vi "add id.vi"(8 "error in (no error)":errorcluster, 10 "id value":variant, 11 "Cluster in":variant) -> (0 "error out":errorcluster, 3 "Cluster out":variant)   [LabVIEW 2017, in "JSONRPC Server.lvclass"]
uses:
  JSONRPC Server.lvclass
  <vilib>/National Instruments/Variant Data Manipulation/Insert Element at End.vi
  <vilib>/National Instruments/Variant Data Manipulation/Variant Data Manipulation.lvlib
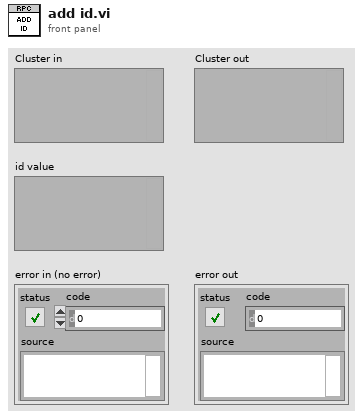
[diagram p1: front panel]
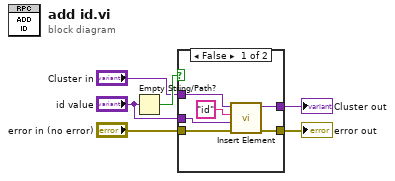
[diagram p0: block diagram]
diagram:
  n1 = Empty String/Path?(string/path="id value") -> (empty?=w5:bool)
  n2 = case shown="False" w5 {
    tunnel: "Cluster in" -> [w12 w14]
    tunnel: [w10 w14] -> w2
    tunnel: [w9 w13] -> w3
    tunnel: "error in (no error)" -> [w8 w13]
    tunnel: "id value" -> [w7 _]
    frame False {
      n3 = call-poly <vilib>:"Insert Element.vi"("error in (no error)"=w8, "element"=w7, "Name"="id", "Cluster in"=w12) -> ("error out"=w9:errorcluster, "Cluster out"=w10:variant)  [unwired: 6 in]
    }
    frame True {
    }
  }
  "error out" <- w3
  "Cluster out" <- w2
